vi "Valide Slave.vi"(8 "error in (no error)":errorcluster, 11 "motor slave info in":T1 {"nodeAddr" format="%.0x"}) -> (0 "error out":errorcluster, 2 "valid?":bool, 3 "motor slave info out":T1 {"nodeAddr" format="%.0x"})   [LabVIEW 2017, in "NI_Robotics_KUKA youBot Host.lvlib"]
uses:
  <vilib>/robotics/KUKA youBot/NI_Robotics_KUKA youBot Host.lvlib
  <vilib>/robotics/KUKA youBot/EtherCAT/Motor Slave Info.ctl
  <vilib>/robotics/KUKA youBot/EtherCAT/LowLevel/Mater Handler.ctl
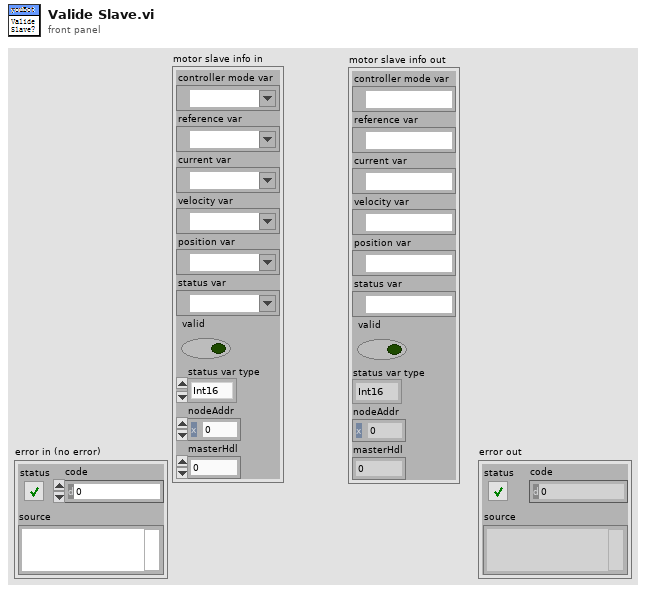
[diagram p1: front panel]
types:
  T1 = typedef "NI_Robotics_KUKA youBot Host.lvlib/Motor Slave Info.ctl" = cluster{"controller mode var":refnum<k21>, "reference var":refnum<k21>, "current var":refnum<k21>, "velocity var":refnum<k21>, "position var":refnum<k21>, "status var":refnum<k21>, "valid":bool, "status var type":enum16{"Int16", "Int32"}, "nodeAddr":u16, "masterHdl":T2}
  T2 = typedef "NI_Robotics_KUKA youBot Host.lvlib/Mater Handler.ctl" = i32
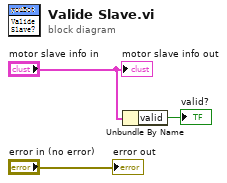
[diagram p0: block diagram]
diagram:
  n1 = Unbundle By Name("motor slave info in") -> ("valid"=→"valid?":bool)
  "error out" <- "error in (no error)"
  "motor slave info out" <- "motor slave info in"
